vi "Parse 1553 xml with owl utils.vi"() -> ()   [LabVIEW 2011]
uses:
  1553 Xfer Info.ctl
  1553 RT Info.ctl
  <instrlib>/AIT 1553/Public/AIT 1553 Controls/Xfer Direction.ctl
  <userlib>/MIL-STD-1553/Owl1553.lvlib
  <userlib>/ARINC-429/Owl429.lvlib
  <instrlib>/AIT 1553/AIT 1553.lvlib
panel:
  out "RT Rx Array":T1[](array[typedef])
  out "RT Tx Array":T1[](array[typedef])
  out "RT Rx Array":bool[][](array[boolean])
  out "RT Tx Array":bool[][](array[boolean])
  out "BM Rx Array":bool[][](array[boolean])
  out "BM Tx Array":bool[][](array[boolean])
  out "BC Array":T3[](array[typedef])
  out "BC Sizes":u32[](array[numeric])
  out "BC Initial Buffer Data":u16[][](array[numeric]) format="%.0x"
  out "buffer count":u32
  out "minor frame count":u32
  out "error out":errorcluster
  out "bus protocol":T4(ring)
  in  "Path in":path=path "C:/work/SE/Opportunities/2012/Pilatus/201210/TestXMLs/Receiver.xml"
  in  "board config handle":u32
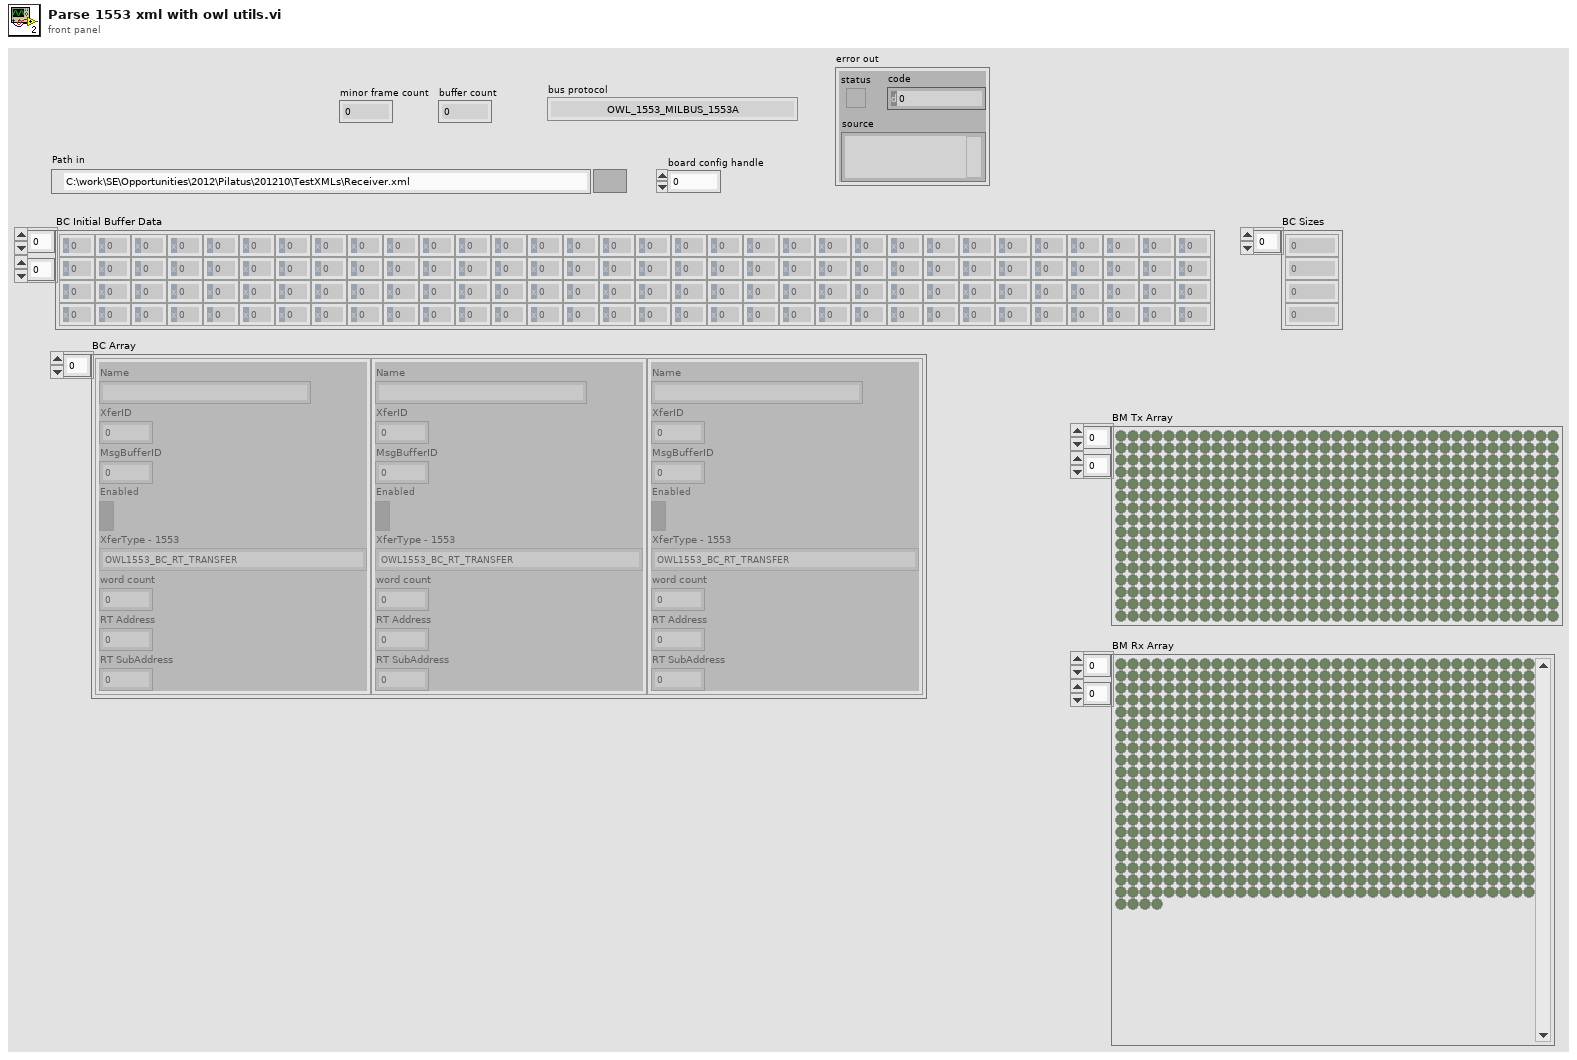
[diagram p1: front panel]
types:
  T1 = typedef "1553 RT Info.ctl" = cluster{"sub address":u8, "transfer direction":T2, "transfer handle out":u32}
  T2 = typedef "AIT 1553.lvlib/Xfer Direction.ctl" = enum16{"RECEIVE_TRANSFER", "TRANSMIT_TRANSFER"}
  T3 = typedef "1553 Xfer Info.ctl" = cluster{"Name":string, "XferID":u8, "MsgBufferID":u8, "Enabled":bool, "XferType - 1553":enum16{"OWL1553_BC_RT_TRANSFER", "OWL1553_RT_BC_TRANSFER", "OWL1553_RT_RT_TRANSFER", "OWL1553_STROBE_TRANSFER", "OWL1553_DELAY_TRANSFER"}, "word count":u8, "RT Address":u8, "RT SubAddress":u8}
  T4 = enum16{"OWL_1553_MILBUS_1553A", "OWL_1553_MILBUS_1553B"}
  T5 = enum16{"OWL1553_RECEIVE_TRANSFER", "OWL1553_TRANSMIT_TRANSFER"}
  T6 = enum16{"OWL_1553_MILBUS_CHANNEL_PRIMARY", "OWL_1553_MILBUS_CHANNEL_SECONDARY"}
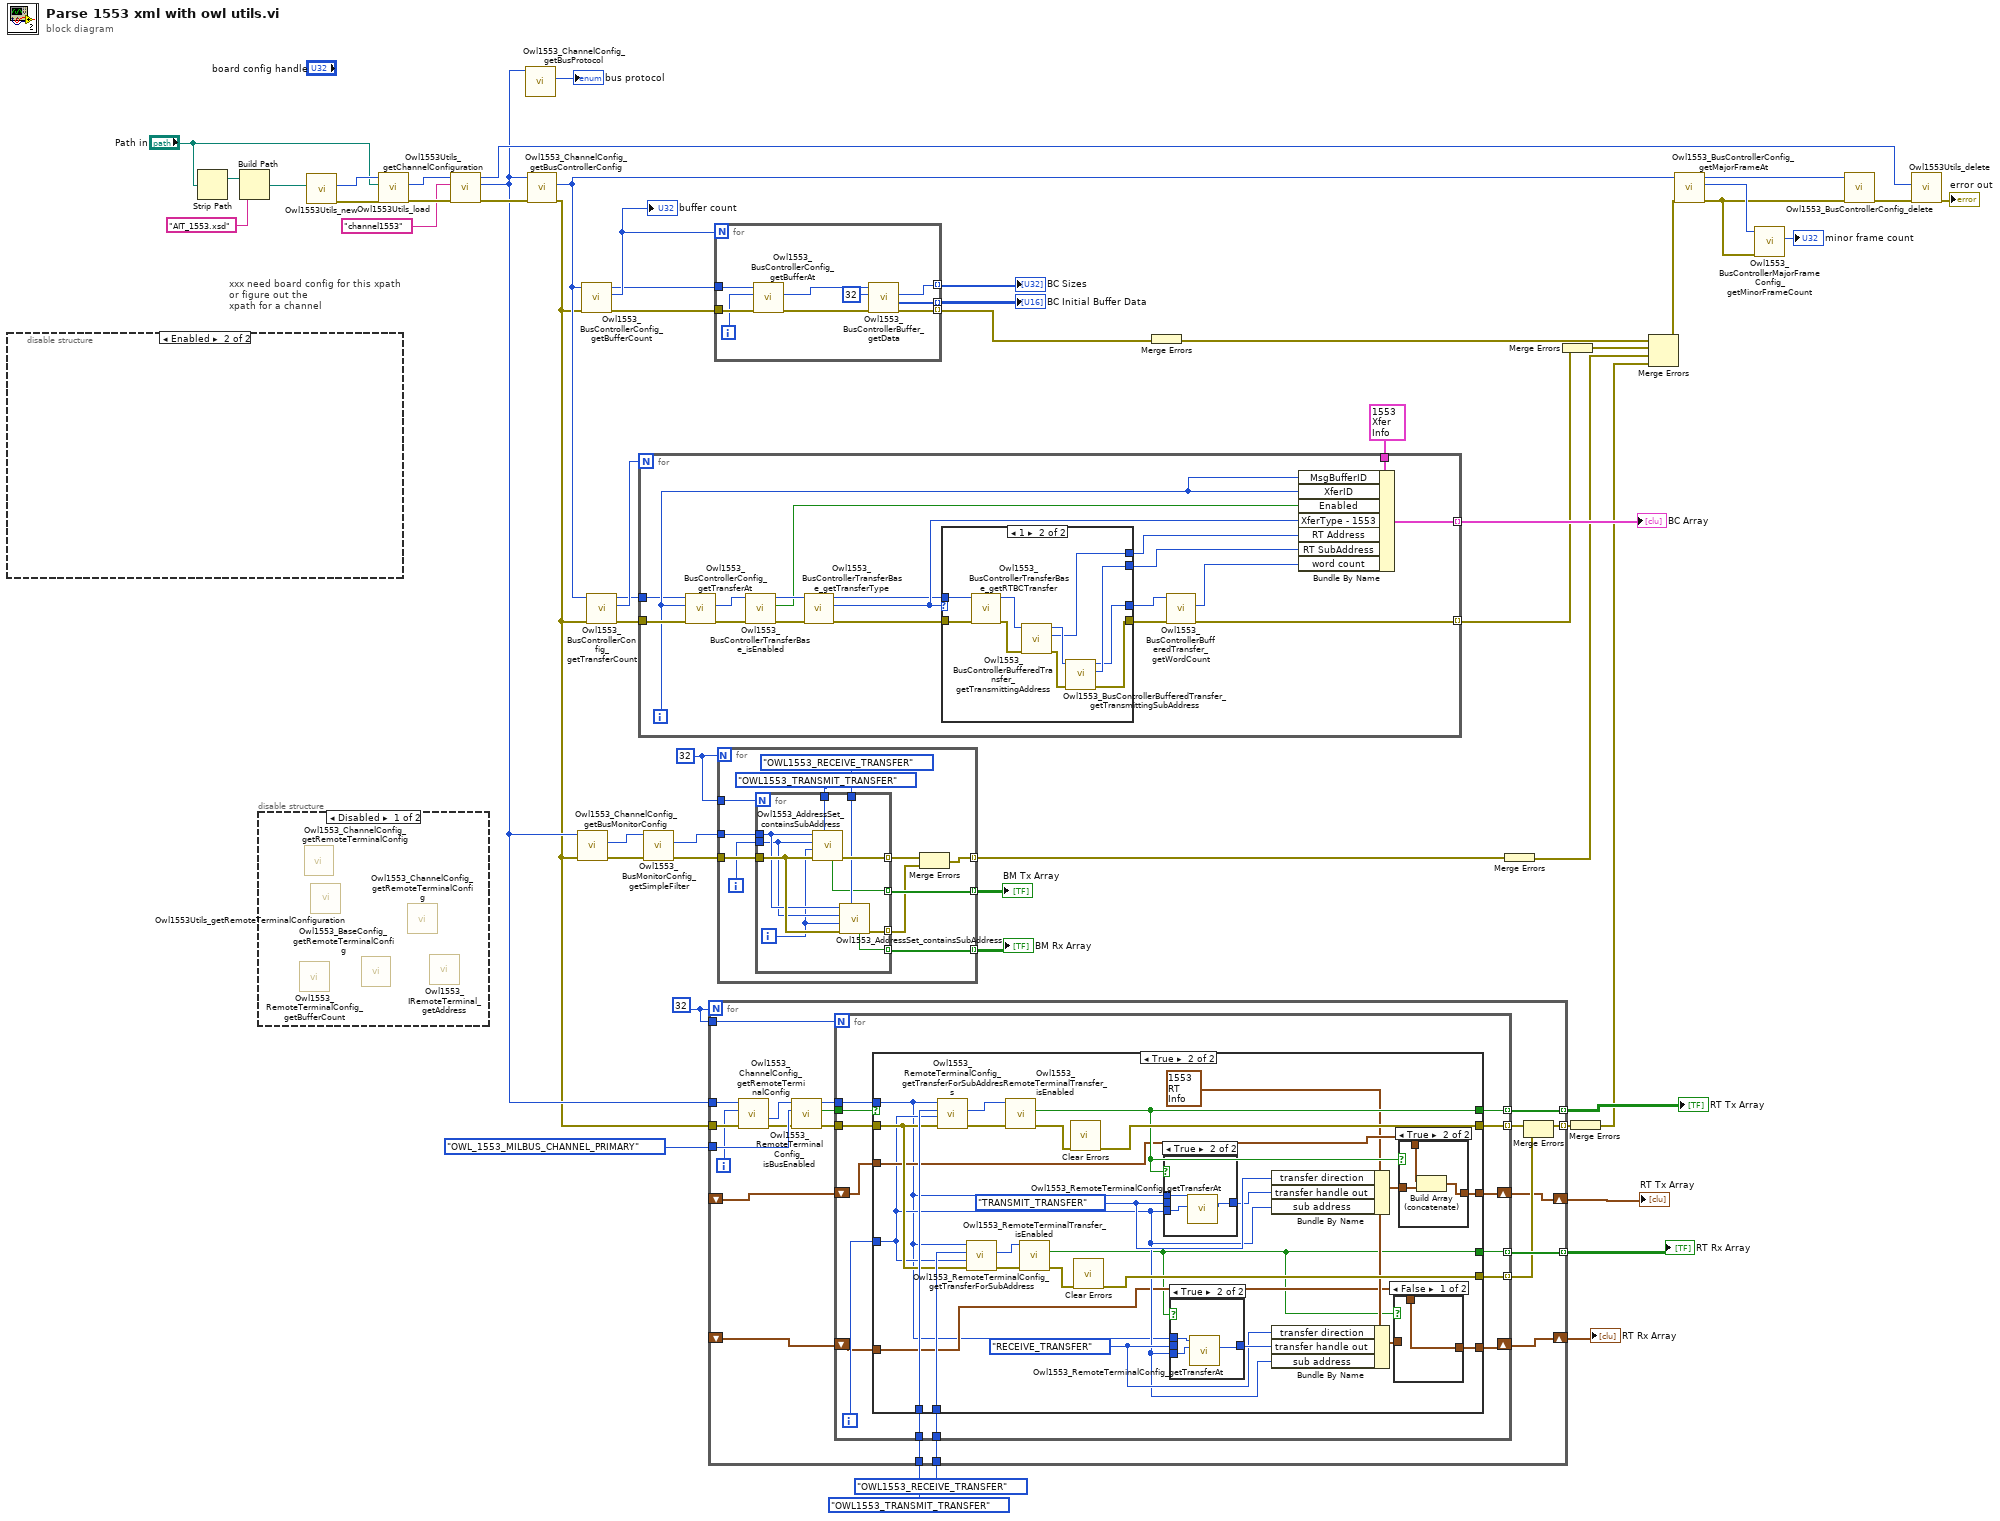
[diagram p0: block diagram]
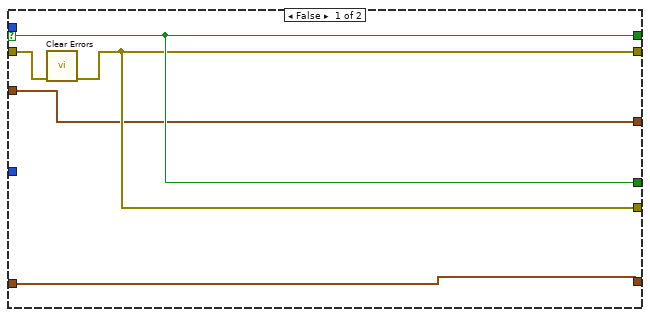
[diagram p3: hidden frame]
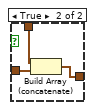
[diagram p4: hidden frame]
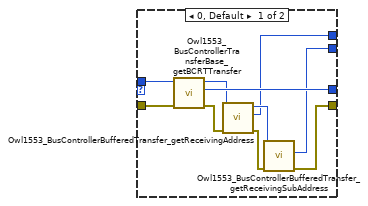
[diagram p8: hidden frame]
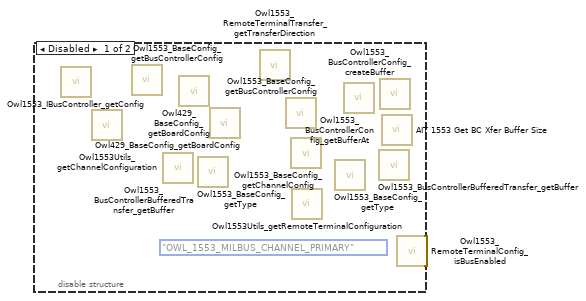
[diagram p9: hidden frame]
diagram:
  w12 = 32
  w16 = 32
  # "xxx need board config for this xpath\nor figure out the\nxpath for a channel"
  n1 = disable-structure shown="Enabled" {
    frame Disabled {
      (unwired) T6."OWL_1553_MILBUS_CHANNEL_PRIMARY" ("milbus")
      n2 = call <userlib>:"Owl1553_IBusController_getConfig.vi"() -> ()  [unwired: 9 in, 3 out]
      n3 = call <userlib>:"Owl1553Utils_getChannelConfiguration.vi"() -> ()  [unwired: 9 in, 3 out]
      n4 = call <userlib>:"Owl1553_BaseConfig_getBusControllerConfig.vi"() -> ()  [unwired: 9 in, 3 out]
      n5 = call <userlib>:"Owl1553_BusControllerBufferedTransfer_getBuffer.vi"() -> ()  [unwired: 8 in, 3 out]
      n6 = call <userlib>:"Owl429_BaseConfig_getBoardConfig.vi"() -> ()  [unwired: 9 in, 3 out]
      n7 = call <userlib>:"Owl1553_BaseConfig_getType.vi"() -> ()  [unwired: 9 in, 3 out]
      n8 = call <userlib>:"Owl429_BaseConfig_getBoardConfig.vi"() -> ()  [unwired: 9 in, 3 out]
      n9 = call <userlib>:"Owl1553_RemoteTerminalTransfer_getTransferDirection.vi"() -> ()  [unwired: 9 in, 3 out]
      n10 = call <userlib>:"Owl1553_BaseConfig_getBusControllerConfig.vi"() -> ()  [unwired: 9 in, 3 out]
      n11 = call <userlib>:"Owl1553_BaseConfig_getChannelConfig.vi"() -> ()  [unwired: 9 in, 3 out]
      n12 = call <userlib>:"Owl1553Utils_getRemoteTerminalConfiguration.vi"() -> ()  [unwired: 9 in, 3 out]
      n13 = call <userlib>:"Owl1553_BaseConfig_getType.vi"() -> ()  [unwired: 9 in, 3 out]
      n14 = call <userlib>:"Owl1553_BusControllerConfig_getBufferAt.vi"() -> ()  [unwired: 9 in, 3 out]
      n15 = call <userlib>:"Owl1553_BusControllerBufferedTransfer_getBuffer.vi"() -> ()  [unwired: 8 in, 3 out]
      n16 = call <userlib>:"Owl1553_BusControllerConfig_createBuffer.vi"() -> ()  [unwired: 9 in, 3 out]
      n17 = call <instrlib>:"AIT 1553 Get BC Xfer Buffer Size.vi"() -> ()  [unwired: 9 in, 3 out]
      n18 = call <userlib>:"Owl1553_RemoteTerminalConfig_isBusEnabled.vi"() -> ()  [unwired: 9 in, 3 out]
    }
    frame Enabled {
    }
  }
  n19 = Strip Path(path="Path in") -> (stripped path=w51:path)  [unwired: 1 out]
  n20 = Build Path(base path=w51, name or relative path="AIT_1553.xsd") -> (appended path=w49:path)
  n21 = disable-structure shown="Disabled" {
    frame Disabled {
      n22 = call <userlib>:"Owl1553_RemoteTerminalConfig_getBufferCount.vi"() -> ()  [unwired: 9 in, 3 out]
      n23 = call <userlib>:"Owl1553_ChannelConfig_getRemoteTerminalConfig.vi"() -> ()  [unwired: 8 in, 4 out]
      n24 = call <userlib>:"Owl1553Utils_getRemoteTerminalConfiguration.vi"() -> ()  [unwired: 9 in, 3 out]
      n25 = call <userlib>:"Owl1553_BaseConfig_getRemoteTerminalConfig.vi"() -> ()  [unwired: 9 in, 3 out]
      n26 = call <userlib>:"Owl1553_ChannelConfig_getRemoteTerminalConfig.vi"() -> ()  [unwired: 8 in, 4 out]
      n27 = call <userlib>:"Owl1553_IRemoteTerminal_getAddress.vi"() -> ()  [unwired: 9 in, 3 out]
    }
    frame Enabled {
    }
  }
  n28 = call <userlib>:"Owl1553Utils_new.vi"("Xml Schema Path in"=w49) -> ("error out"=w54:errorcluster, "xml config handle"=w48:u32)  [unwired: 9 in]
  n29 = call <userlib>:"Owl1553Utils_load.vi"("error in (no error)"=w54, "Path in"="Path in", "xml config handle"=w48) -> ("error out"=w53:errorcluster, "xml config handle"=w52:u32)  [unwired: 7 in]
  n30 = call <userlib>:"Owl1553Utils_getChannelConfiguration.vi"("error in (no error)"=w53, "X Path"="channel1553", "xml config handle"=w52) -> ("error out"=w55:errorcluster, "channel config handle"=w14:u32, "xml config handle"=w44:u32)  [unwired: 6 in]
  n31 = call <userlib>:"Owl1553_ChannelConfig_getBusProtocol.vi"("channel config handle"=w14) -> ("bus protocol"=→"bus protocol":T4)  [unwired: 8 in, 2 out]
  n32 = call <userlib>:"Owl1553_ChannelConfig_getBusControllerConfig.vi"("error in (no error)"=w55, "channel config handle"=w14) -> ("error out"=w13:errorcluster, "bus controller config handle"=w31:u32)  [unwired: 7 in, 1 out]
  n33 = call <userlib>:"Owl1553_ChannelConfig_getBusMonitorConfig.vi"("error in (no error)"=w13, "channel config handle"=w14) -> ("error out"=w23:errorcluster, "bus monitor config handle"=w24:u32)  [unwired: 7 in, 1 out]
  n34 = call <userlib>:"Owl1553_BusControllerConfig_getBufferCount.vi"("error in (no error)"=w13, "bus controller config handle"=w31) -> ("error out"=w35:errorcluster, "buffer count"=w37:u32, "bus controller config handle"=w36:u32)  [unwired: 7 in]
  "buffer count" <- w37
  n35 = call <userlib>:"Owl1553_BusControllerConfig_getTransferCount.vi"("error in (no error)"=w13, "bus controller config handle"=w31) -> ("error out"=w28:errorcluster, "transfer count"=w30:u32, "bus controller config handle"=w29:u32)  [unwired: 7 in]
  n36 = for {
    N: w30 -> [_]
    tunnel: w29 -> [w58]
    tunnel: w28 -> [w74]
    tunnel: [w67] -> w27 mode=indexing
    tunnel: T3 {"Name"="", "XferID"=0, "MsgBufferID"=0, "Enabled"=FALSE, "XferType - 1553"=enum."OWL1553_BC_RT_TRANSFER", "word count"=0, "RT Address"=0, "RT SubAddress"=0} ("XferInfo") -> [w66]
    tunnel: [w61] -> w26 mode=indexing
    i -> [w60]
    n37 = call <userlib>:"Owl1553_BusControllerConfig_getTransferAt.vi"("error in (no error)"=w74, "index"=w60, "bus controller config handle"=w58) -> ("error out"=w59:errorcluster, "transfer base handle"=w56:u32)  [unwired: 6 in, 1 out]
    n38 = call <userlib>:"Owl1553_BusControllerTransferBase_isEnabled.vi"("error in (no error)"=w59, "transferbase handle"=w56) -> ("error out"=w71:errorcluster, "enabled"=w69:bool, "transferbase handle"=w70:u32)  [unwired: 6 in]
    n39 = call <userlib>:"Owl1553_BusControllerTransferBase_getTransferType.vi"("error in (no error)"=w71, "transferbase handle"=w70) -> ("error out"=w72:errorcluster, "transfer type"=w68:i32, "transferbase handle"=w57:u32)  [unwired: 6 in]
    n40 = case shown="1" w68 {
      tunnel: w72 -> [w84 w94]
      tunnel: [w75 w85] -> w73
      tunnel: [w83 w86] -> w65
      tunnel: w57 -> [w82 w93]
      tunnel: [w77 w88] -> w64
      tunnel: [w76 w87] -> w63
      frame 0, Default {
        n41 = call <userlib>:"Owl1553_BusControllerTransferBase_getBCRTTransfer.vi"("error in (no error)"=w84, "transferbase handle"=w82) -> ("error out"=w81:errorcluster, "bcrt transfer handle"=w83:u32, "transferbase handle"=w79:u32)  [unwired: 6 in]
        n42 = call <userlib>:"Owl1553_BusControllerBufferedTransfer_getReceivingAddress.vi"("error in (no error)"=w81, "buffered transfer handle"=w79) -> ("error out"=w80:errorcluster, "remote terminal address"=w77:u8, "buffered transfer handle"=w78:u32)  [unwired: 6 in]
        n43 = call <userlib>:"Owl1553_BusControllerBufferedTransfer_getReceivingSubAddress.vi"("error in (no error)"=w80, "buffered transfer handle"=w78) -> ("error out"=w75:errorcluster, "remote terminal address"=w76:u8)  [unwired: 6 in, 1 out]
      }
      frame 1 {
        n44 = call <userlib>:"Owl1553_BusControllerTransferBase_getRTBCTransfer.vi"("error in (no error)"=w94, "transferbase handle"=w93) -> ("error out"=w91:errorcluster, "transferbase handle"=w92:u32)  [unwired: 6 in, 1 out]
        n45 = call <userlib>:"Owl1553_BusControllerBufferedTransfer_getTransmittingAddress.vi"("error in (no error)"=w91, "buffered transfer handle"=w92) -> ("error out"=w90:errorcluster, "remote terminal address"=w88:u8, "buffered transfer handle"=w89:u32)  [unwired: 6 in]
        n46 = call <userlib>:"Owl1553_BusControllerBufferedTransfer_getTransmittingSubAddress.vi"("error in (no error)"=w90, "buffered transfer handle"=w89) -> ("error out"=w85:errorcluster, "remote terminal sub-address"=w87:u8, "buffered transfer handle"=w86:u32)  [unwired: 6 in]
      }
    }
    n47 = call <userlib>:"Owl1553_BusControllerBufferedTransfer_getWordCount.vi"("error in (no error)"=w73, "buffered transfer handle"=w65) -> ("error out"=w61:errorcluster, "word count"=w62:u8)  [unwired: 6 in, 1 out]
    n48 = Bundle By Name(cluster=w66, "MsgBufferID"=w60, "XferID"=w60, "Enabled"=w69, "XferType - 1553"=w68, "RT Address"=w64, "RT SubAddress"=w63, "word count"=w62) -> (w67:T3)
  }
  "BC Array" <- w27
  n49 = call <userlib>:"Owl1553_BusMonitorConfig_getSimpleFilter.vi"("error in (no error)"=w23, "config handle"=w24) -> ("error out"=w21:errorcluster, "address set handle"=w22:u32)  [unwired: 7 in, 1 out]
  n50 = for {
    N: w12 -> [_]
    tunnel: T6."OWL_1553_MILBUS_CHANNEL_PRIMARY" ("milbus") -> [w114]
    tunnel: [w100] -> w15 mode=indexing
    tunnel: w14 -> [w115]
    tunnel: w13 -> [w111]
    tunnel: w12 -> [w106]
    tunnel: [w105] -> w11 mode=indexing
    tunnel: T5."OWL1553_TRANSMIT_TRANSFER" ("direction") -> [w103]
    tunnel: T5."OWL1553_RECEIVE_TRANSFER" ("direction") -> [w102]
    tunnel: [w101] -> w9 mode=indexing
    shift-right: [w98] -> w3
    shift-left: _ -> [w97]
    shift-right: [w95] -> w2
    shift-left: _ -> [w96]
    i -> [w110]
    n51 = call <userlib>:"Owl1553_ChannelConfig_getRemoteTerminalConfig.vi"("error in (no error)"=w111, "remote terminal"=w110, "channel config handle"=w115) -> ("error out"=w113:errorcluster, "remote terminal config handle"=w112:u32)  [unwired: 5 in, 2 out]
    n52 = call <userlib>:"Owl1553_RemoteTerminalConfig_isBusEnabled.vi"("error in (no error)"=w113, "milbus"=w114, "remote terminal config handle"=w112) -> ("error out"=w109:errorcluster, "is enabled"=w107:bool, "remote terminal config handle"=w104:u32)  [unwired: 6 in]
    n53 = for {
      N: w106 -> [_]
      tunnel: [w126] -> w108 mode=indexing
      tunnel: w109 -> [w129]
      tunnel: w107 -> [w128]
      tunnel: [w127] -> w105 mode=indexing
      tunnel: w104 -> [w125]
      tunnel: w103 -> [w123]
      tunnel: w102 -> [w122]
      tunnel: [w121] -> w101 mode=indexing
      tunnel: [w120] -> w99 mode=indexing
      shift-right: [w119] -> w98
      shift-left: w97 -> [w118]
      shift-right: [w116] -> w95
      shift-left: w96 -> [w117]
      i -> [w124]
      n54 = case shown="True" w128 {
        selector: w128 -> [w134 _]
        tunnel: [w132 w154] -> w126
        tunnel: w129 -> [w133 w156]
        tunnel: [w134 w149] -> w127
        tunnel: w125 -> [_ w135]
        tunnel: w124 -> [_ w143]
        tunnel: w123 -> [_ w160]
        tunnel: w122 -> [_ w159]
        tunnel: [w134 w138] -> w121
        tunnel: [w132 w152] -> w120
        tunnel: [w131 w146] -> w119
        tunnel: w118 -> [w131 w148]
        tunnel: w117 -> [w130 w141]
        tunnel: [w130 w140] -> w116
        frame False {
          n55 = call <vilib>:"Clear Errors.vi"("error in (no error)"=w133) -> ("error out"=w132:errorcluster)  [unwired: 6 in]
        }
        frame True {
          w144 = Xfer_Direction."RECEIVE_TRANSFER" ("direction in")
          w151 = Xfer_Direction."TRANSMIT_TRANSFER" ("direction in")
          w142 = T1 {"sub address"=0, "transfer direction"=enum."RECEIVE_TRANSFER", "transfer handle out"=0} ("RT Item")
          n56 = call <userlib>:"Owl1553_RemoteTerminalConfig_getTransferForSubAddress.vi"("error in (no error)"=w156, "sub address"=w143, "direction"=w160, "remote terminal config handle"=w135) -> ("error out"=w158:errorcluster, "transfer handle"=w137:u32)  [unwired: 5 in, 1 out]
          n57 = call <userlib>:"Owl1553_RemoteTerminalConfig_getTransferForSubAddress.vi"("error in (no error)"=w156, "sub address"=w143, "direction"=w159, "remote terminal config handle"=w135) -> ("error out"=w157:errorcluster, "transfer handle"=w136:u32)  [unwired: 5 in, 1 out]
          n58 = call <userlib>:"Owl1553_RemoteTerminalTransfer_isEnabled.vi"("error in (no error)"=w158, "remote terminal transfer handle"=w137) -> ("error out"=w155:errorcluster, "is enabled"=w149:bool)  [unwired: 7 in, 1 out]
          n59 = call <userlib>:"Owl1553_RemoteTerminalTransfer_isEnabled.vi"("error in (no error)"=w157, "remote terminal transfer handle"=w136) -> ("error out"=w153:errorcluster, "is enabled"=w138:bool)  [unwired: 7 in, 1 out]
          n60 = call <vilib>:"Clear Errors.vi"("error in (no error)"=w155) -> ("error out"=w154:errorcluster)  [unwired: 6 in]
          n61 = call <vilib>:"Clear Errors.vi"("error in (no error)"=w153) -> ("error out"=w152:errorcluster)  [unwired: 6 in]
          n62 = case shown="True" w149 {
            tunnel: w151 -> [_ _]
            tunnel: w135 -> [_ w174]
            tunnel: w143 -> [_ w173]
            tunnel: [_ w172] -> w150
            frame False {
            }
            frame True {
              n63 = call <userlib>:"Owl1553_RemoteTerminalConfig_getTransferAt.vi"("index"=w173, "remote terminal config handle"=w174) -> ("transfer handle"=w172:u32)  [unwired: 7 in, 2 out]
            }
          }
          n64 = case shown="True" w138 {
            tunnel: w144 -> [_ _]
            tunnel: w135 -> [_ w167]
            tunnel: w143 -> [_ w166]
            tunnel: [_ w165] -> w145
            frame False {
            }
            frame True {
              n65 = call <userlib>:"Owl1553_RemoteTerminalConfig_getTransferAt.vi"("index"=w166, "remote terminal config handle"=w167) -> ("transfer handle"=w165:u32)  [unwired: 7 in, 2 out]
            }
          }
          n66 = Bundle By Name(cluster=w142, "transfer direction"=w151, "transfer handle out"=w150, "sub address"=w143) -> (w147:T1)
          n67 = Bundle By Name(cluster=w142, "transfer direction"=w144, "transfer handle out"=w145, "sub address"=w143) -> (w139:T1)
          n68 = case shown="False" w138 {
            tunnel: w141 -> [w161 w164]
            tunnel: w139 -> [_ w163]
            tunnel: [w161 w162] -> w140
            frame False {
            }
            frame True {
              n69 = Build Array (concatenate)(w164, w163) -> (w162:T1[])
            }
          }
          n70 = case shown="True" w149 {
            tunnel: w148 -> [w168 w171]
            tunnel: w147 -> [_ w170]
            tunnel: [w168 w169] -> w146
            frame False {
            }
            frame True {
              n71 = Build Array (concatenate)(w171, w170) -> (w169:T1[])
            }
          }
        }
      }
    }
    n72 = Merge Errors(w108, w99) -> (w100:errorcluster)
  }
  "RT Tx Array" <- w11
  "RT Rx Array" <- w9
  "RT Tx Array" <- w3
  "RT Rx Array" <- w2
  n73 = for {
    N: w37 -> [_]
    tunnel: w36 -> [w183]
    tunnel: w35 -> [w182]
    tunnel: [w180] -> w34 mode=indexing
    tunnel: [w179] -> w33 mode=indexing
    tunnel: [w178] -> w25 mode=indexing
    i -> [w181]
    n74 = call <userlib>:"Owl1553_BusControllerConfig_getBufferAt.vi"("error in (no error)"=w182, "index"=w181, "bus controller config handle"=w183) -> ("error out"=w177:errorcluster, "buffer handle"=w176:u32)  [unwired: 6 in, 1 out]
    n75 = call <userlib>:"Owl1553_BusControllerBuffer_getData.vi"("error in (no error)"=w177, "buffer size"=u32 32, "bus controller buffer handle"=w176) -> ("error out"=w178:errorcluster, "data"=w180:u16[], "buffer size out"=w179:u32)  [unwired: 5 in, 1 out]
  }
  "BC Initial Buffer Data" <- w34
  "BC Sizes" <- w33
  n76 = for {
    N: w16 -> [_]
    tunnel: w22 -> [w194]
    tunnel: w21 -> [w193]
    tunnel: [w190] -> w20 mode=indexing
    tunnel: [w191] -> w19 mode=indexing
    tunnel: w16 -> [w188]
    tunnel: [w184] -> w18 mode=indexing
    i -> [w189]
    n77 = for {
      N: w188 -> [_]
      tunnel: w194 -> [w201]
      tunnel: w193 -> [w202]
      tunnel: [w197] -> w191 mode=indexing
      tunnel: [w204] -> w192 mode=indexing
      tunnel: w189 -> [w200]
      tunnel: [w203] -> w187 mode=indexing
      tunnel: T5."OWL1553_TRANSMIT_TRANSFER" ("direction") -> [w195]
      tunnel: T5."OWL1553_RECEIVE_TRANSFER" ("direction") -> [w198]
      tunnel: [w196] -> w184 mode=indexing
      i -> [w199]
      n78 = call <userlib>:"Owl1553_AddressSet_containsSubAddress.vi"("direction"=w195, "error in (no error)"=w202, "sub address"=w199, "remote terminal address"=w200, "address set handle"=w201) -> ("error out"=w204:errorcluster, "contains sub-address"=w197:bool)  [unwired: 4 in, 1 out]
      n79 = call <userlib>:"Owl1553_AddressSet_containsSubAddress.vi"("direction"=w198, "error in (no error)"=w202, "sub address"=w199, "remote terminal address"=w200, "address set handle"=w201) -> ("error out"=w203:errorcluster, "contains sub-address"=w196:bool)  [unwired: 4 in, 1 out]
    }
    n80 = Merge Errors(w192, w187) -> (w190:errorcluster)
  }
  "BM Tx Array" <- w19
  "BM Rx Array" <- w18
  n81 = Merge Errors(w25) -> (w7:errorcluster)
  n82 = Merge Errors(w20) -> (w5:errorcluster)
  n83 = Merge Errors(w26) -> (w6:errorcluster)
  n84 = Merge Errors(w15) -> (w4:errorcluster)
  n85 = Merge Errors(w7, w6, w5, w4) -> (w32:errorcluster)
  n86 = call <userlib>:"Owl1553_BusControllerConfig_getMajorFrameAt.vi"("error in (no error)"=w32, "bus controller config handle"=w31) -> ("error out"=w38:errorcluster, "major frame config handle"=w40:u32, "bus controller config handle"=w45:u32)  [unwired: 7 in]
  n87 = call <userlib>:"Owl1553_BusControllerMajorFrameConfig_getMinorFrameCount.vi"("error in (no error)"=w38, "config handle"=w40) -> ("minor frame count"=→"minor frame count":u32)  [unwired: 7 in, 2 out]
  n88 = call <userlib>:"Owl1553_BusControllerConfig_delete.vi"("error in (no error)"=w38, "bus controller config handle"=w45) -> ("error out"=w46:errorcluster)  [unwired: 9 in]
  n89 = call <userlib>:"Owl1553Utils_delete.vi"("error in (no error)"=w46, "xml config handle"=w44) -> ("error out"=→"error out":errorcluster)  [unwired: 9 in]
